vi "pathplan.vi"() -> ()   [LabVIEW 2016]
uses:
  <vilib>/imath/engines/lvmath2/RunTimeEngine/NodeEndStatement/NIMS_NodeEndStatement_Output.vi
  <instcachedir>/0/NIMS_NodeEndStatement_Output_53EC0D466D134D7ABD903AC30B43404B.lvgen/NIMS_NodeEndStatement_Output_53EC0D466D134D7ABD903AC30B43404B_011.vi
  <vilib>/imath/engines/lvmath2/RunTimeEngine/ErrorHandling/NIMS_Finalize Error.vi
panel:
  out "起点监视2":sgl[](array[numeric])
  in  "目标位置2":dbl[](array[numeric])=[6000.0, 1500.0]
  out "起点监视3":sgl[](array[numeric])
  in  "目标位置3":dbl[](array[numeric])=[2645.0, 2645.0]
  out "起点监视0":sgl[](array[numeric])
  in  "目标位置0":dbl[](array[numeric])=[12000.0, 0.0]
  out "Key1（移动5）":bool
  in  "Key2(点3)":bool
  in  "Key1(点2)":bool
  in  "Key0(点1)":bool
  in  "全场定位串口":refnum<visa-resource-name>="ASRL4::INSTR" caption="全场定位模块"
  in  "speed_max":dbl=15000.0
  in  "发送写入":refnum<visa-resource-name>
  in  "车宽的一半":dbl=200.0
  out "起点监视1":sgl[](array[numeric])
  in  "目标位置1":dbl[](array[numeric])=[9355.0, 2645.0]
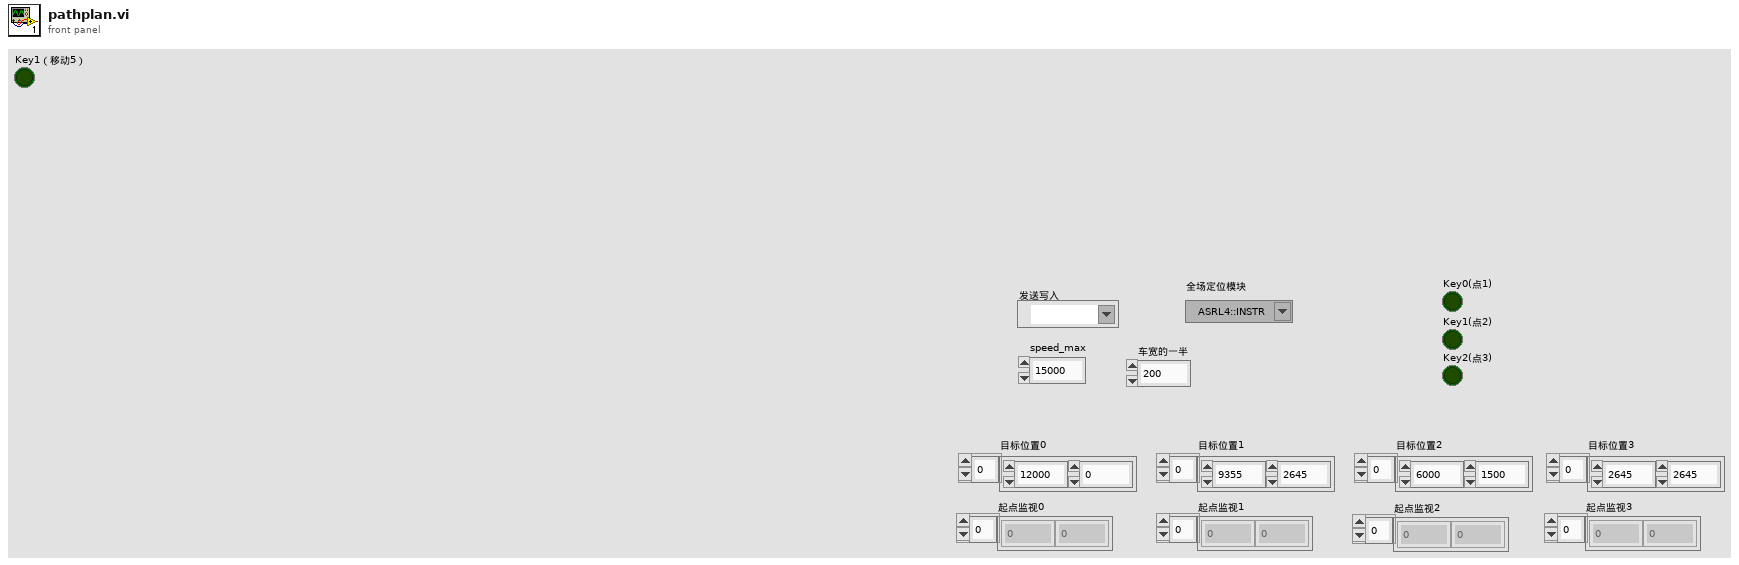
[diagram p1: front panel]
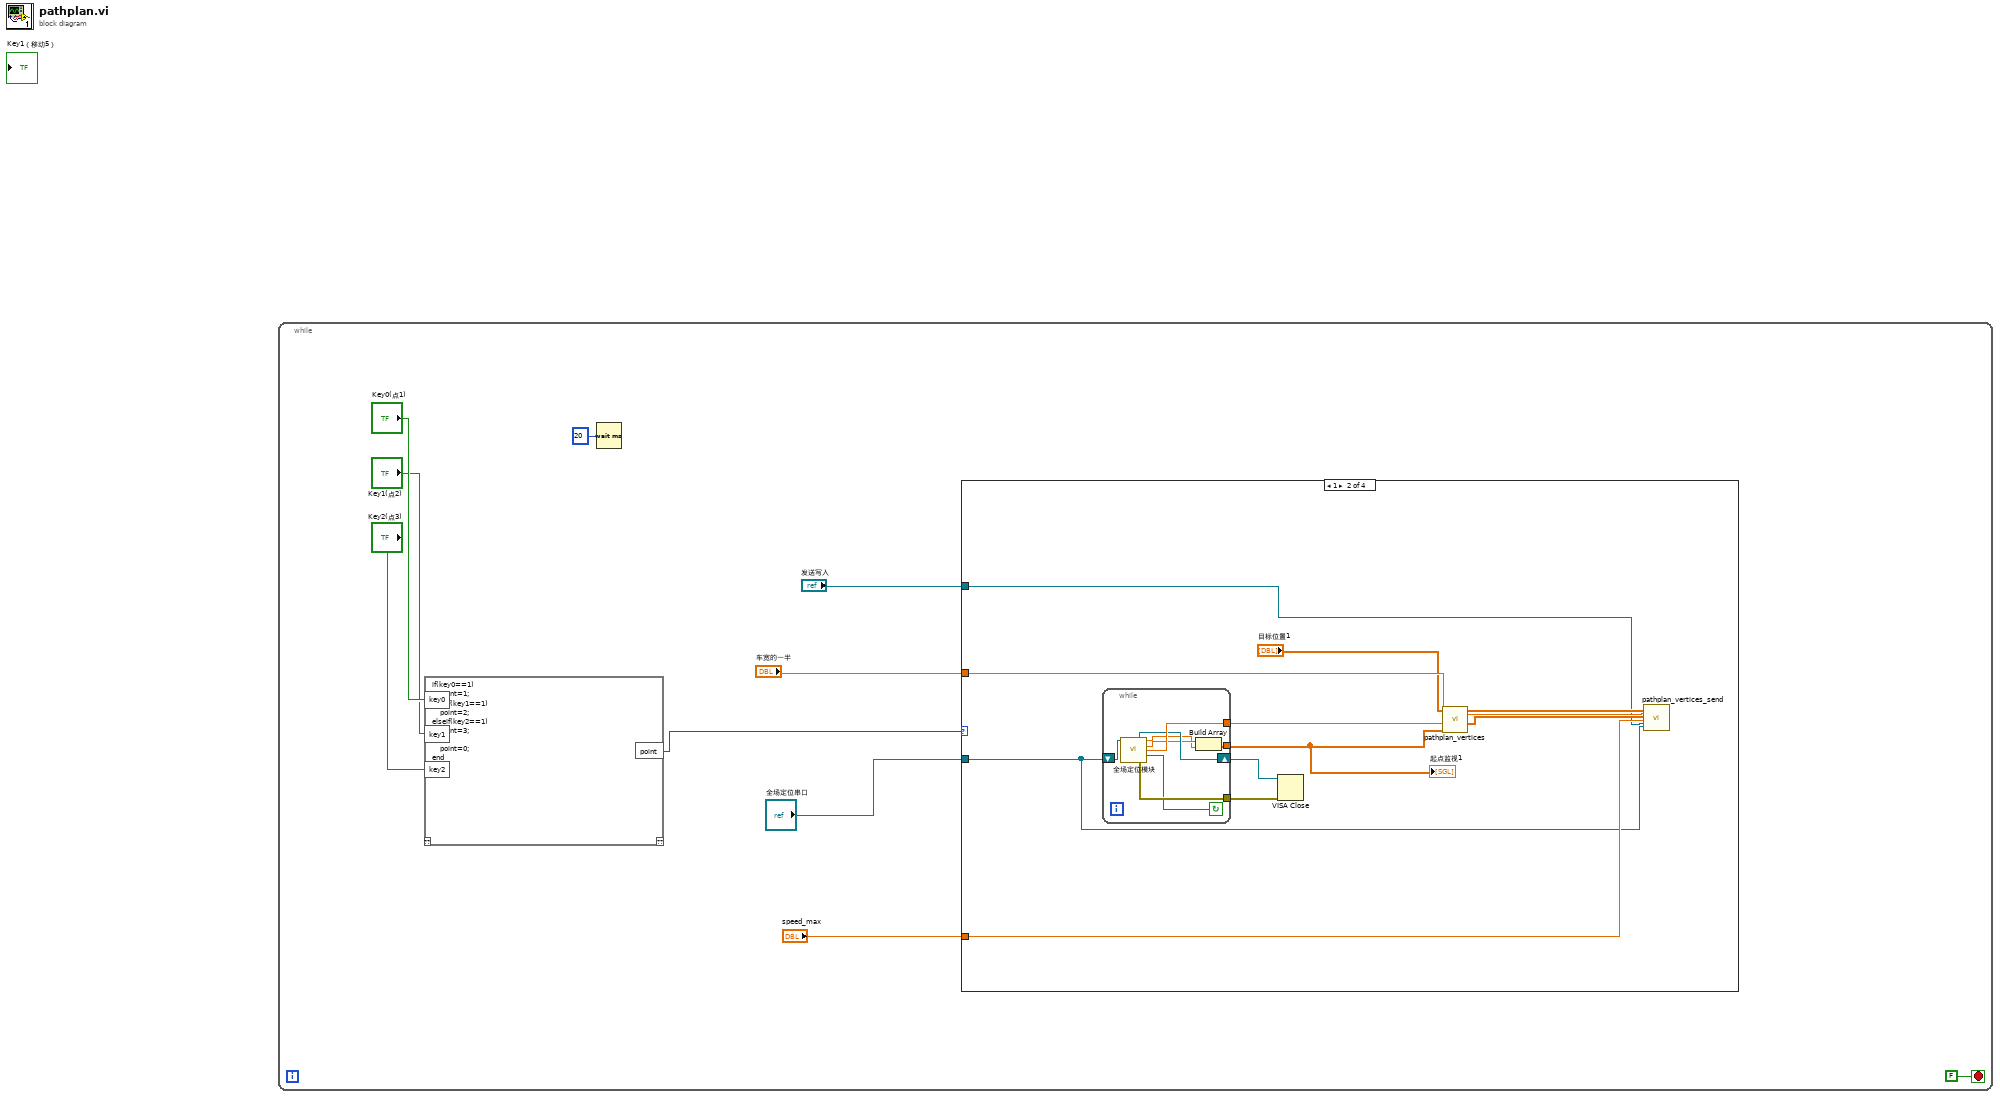
[diagram p0: block diagram]
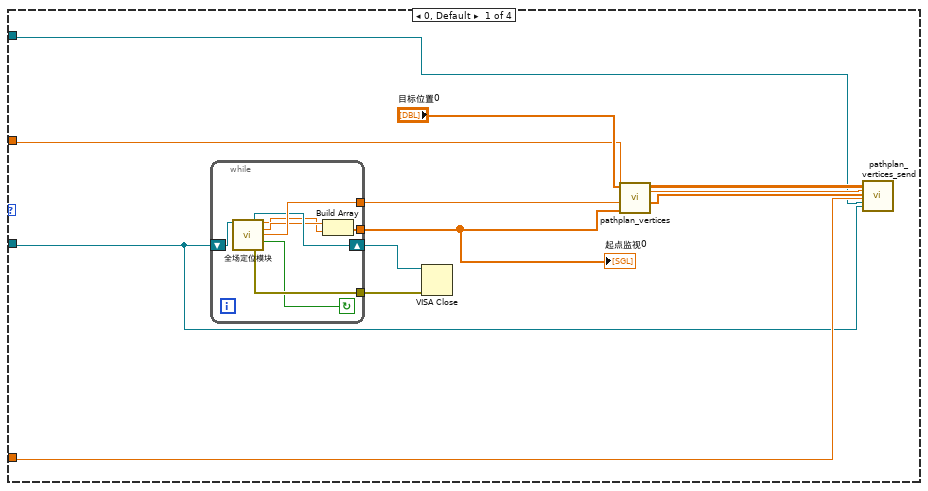
[diagram p2: hidden frame]
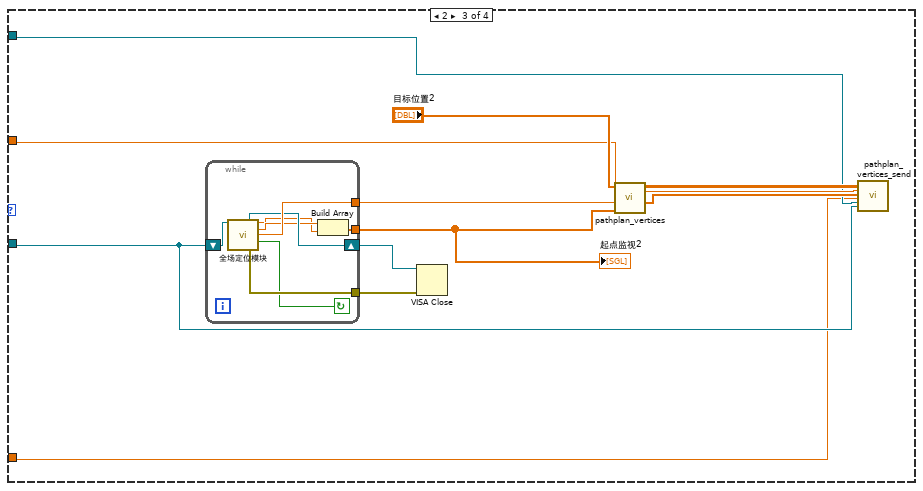
[diagram p3: hidden frame]
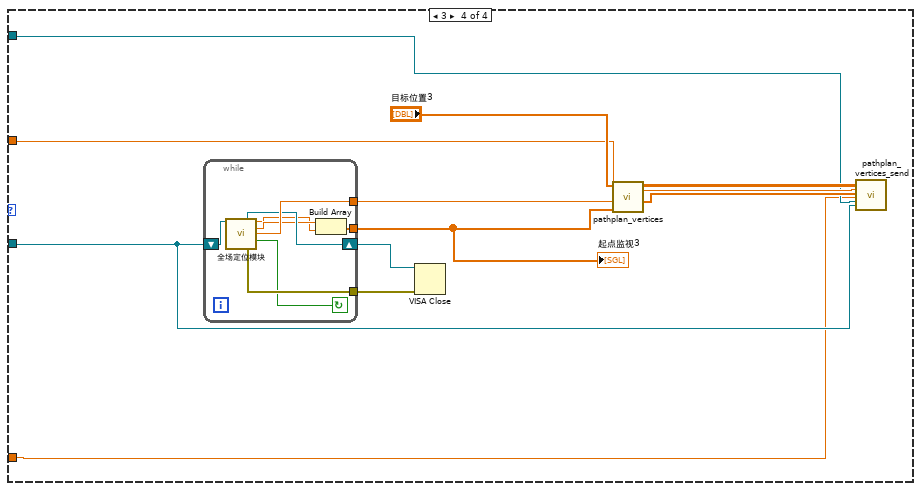
[diagram p4: hidden frame]
diagram:
  n1 = while {
    stop <- FALSE stop-if-true
    n2 = mathscript code="if(key0==1)\n    point=1;\nelseif(key1==1)\n    point=2;\nelseif(key2==1)\n    point=3;\nelse\n    point=0;\nend"("key0"="Key0(点1)", "key1"="Key1(点2)", "key2"="Key2(点3)") -> ("point"=w3:i32)  [unwired: 1 in, 1 out]
    n3 = Wait (ms)(milliseconds to wait=u32 20 ("等待时间（毫秒）")) -> ()  [unwired: 1 out]
    n4 = case shown="1" w3 {
      tunnel: "车宽的一半" -> [w88 w117 w129 w149]
      tunnel: "speed_max" -> [w90 w109 w127 w147]
      tunnel: "发送写入" -> [w87 w108 w130 w150]
      tunnel: "全场定位串口" -> [w89 w107 w128 w148]
      frame 0, Default {
        n5 = while {
          tunnel: [w106] -> w98
          tunnel: [w104] -> w96
          tunnel: [w103] -> w95
          shift-right: [w102] -> w94
          shift-left: w89 -> [w105]
          stop <- w101 continue-if-true
          n6 = call "全场定位模块.vi"("VISA resource name"=w105) -> ("VISA资源名称输出"=w102:refnum<visa-resource-name>, "y"=w99:sgl, "x"=w100:sgl, "Zangle"=w103:sgl, "pd"=w101:bool, "错误输出2"=w104:errorcluster)  [unwired: 8 in, 1 out]
          n7 = Build Array(w100, w99) -> (w106:sgl[])
        }
        "起点监视0" <- w98
        n8 = VISA Close(VISA resource name=w94, error in (no error)=w96) -> ()  [unwired: 1 out]
        n9 = call "pathplan_vertices.vi"("终点"="目标位置0", "车宽的一半"=w88, "z_angle"=w95, "起点"=w98) -> ("vertices"=w93:dbl[][], "distance_all"=w92:dbl, "angle_all"=w91:dbl[])  [unwired: 3 in, 1 out]
        n10 = call "pathplan_vertices_send.vi"("vertices"=w93, "distance_all"=w92, "angle_all"=w91, "speed_max"=w90, "写入串口"=w87, "全场定位"=w89) -> ()  [unwired: 21 in, 1 out]
      }
      frame 1 {
        n11 = while {
          tunnel: [w126] -> w118
          tunnel: [w124] -> w115
          tunnel: [w123] -> w114
          shift-right: [w122] -> w113
          shift-left: w107 -> [w125]
          stop <- w121 continue-if-true
          n12 = call "全场定位模块.vi"("VISA resource name"=w125) -> ("VISA资源名称输出"=w122:refnum<visa-resource-name>, "y"=w119:sgl, "x"=w120:sgl, "Zangle"=w123:sgl, "pd"=w121:bool, "错误输出2"=w124:errorcluster)  [unwired: 8 in, 1 out]
          n13 = Build Array(w120, w119) -> (w126:sgl[])
        }
        "起点监视1" <- w118
        n14 = VISA Close(VISA resource name=w113, error in (no error)=w115) -> ()  [unwired: 1 out]
        n15 = call "pathplan_vertices.vi"("终点"="目标位置1", "车宽的一半"=w117, "z_angle"=w114, "起点"=w118) -> ("vertices"=w112:dbl[][], "distance_all"=w111:dbl, "angle_all"=w110:dbl[])  [unwired: 3 in, 1 out]
        n16 = call "pathplan_vertices_send.vi"("vertices"=w112, "distance_all"=w111, "angle_all"=w110, "speed_max"=w109, "写入串口"=w108, "全场定位"=w107) -> ()  [unwired: 21 in, 1 out]
      }
      frame 2 {
        n17 = while {
          tunnel: [w146] -> w138
          tunnel: [w144] -> w136
          tunnel: [w143] -> w135
          shift-right: [w142] -> w134
          shift-left: w128 -> [w145]
          stop <- w141 continue-if-true
          n18 = call "全场定位模块.vi"("VISA resource name"=w145) -> ("VISA资源名称输出"=w142:refnum<visa-resource-name>, "y"=w139:sgl, "x"=w140:sgl, "Zangle"=w143:sgl, "pd"=w141:bool, "错误输出2"=w144:errorcluster)  [unwired: 8 in, 1 out]
          n19 = Build Array(w140, w139) -> (w146:sgl[])
        }
        "起点监视2" <- w138
        n20 = VISA Close(VISA resource name=w134, error in (no error)=w136) -> ()  [unwired: 1 out]
        n21 = call "pathplan_vertices.vi"("终点"="目标位置2", "车宽的一半"=w129, "z_angle"=w135, "起点"=w138) -> ("vertices"=w133:dbl[][], "distance_all"=w132:dbl, "angle_all"=w131:dbl[])  [unwired: 3 in, 1 out]
        n22 = call "pathplan_vertices_send.vi"("vertices"=w133, "distance_all"=w132, "angle_all"=w131, "speed_max"=w127, "写入串口"=w130, "全场定位"=w128) -> ()  [unwired: 21 in, 1 out]
      }
      frame 3 {
        n23 = while {
          tunnel: [w166] -> w158
          tunnel: [w164] -> w156
          tunnel: [w163] -> w155
          shift-right: [w162] -> w154
          shift-left: w148 -> [w165]
          stop <- w161 continue-if-true
          n24 = call "全场定位模块.vi"("VISA resource name"=w165) -> ("VISA资源名称输出"=w162:refnum<visa-resource-name>, "y"=w159:sgl, "x"=w160:sgl, "Zangle"=w163:sgl, "pd"=w161:bool, "错误输出2"=w164:errorcluster)  [unwired: 8 in, 1 out]
          n25 = Build Array(w160, w159) -> (w166:sgl[])
        }
        "起点监视3" <- w158
        n26 = VISA Close(VISA resource name=w154, error in (no error)=w156) -> ()  [unwired: 1 out]
        n27 = call "pathplan_vertices.vi"("终点"="目标位置3", "车宽的一半"=w149, "z_angle"=w155, "起点"=w158) -> ("vertices"=w153:dbl[][], "distance_all"=w152:dbl, "angle_all"=w151:dbl[])  [unwired: 3 in, 1 out]
        n28 = call "pathplan_vertices_send.vi"("vertices"=w153, "distance_all"=w152, "angle_all"=w151, "speed_max"=w147, "写入串口"=w150, "全场定位"=w148) -> ()  [unwired: 21 in, 1 out]
      }
    }
  }
